vi "Calibration GUI.vi"(8 "error in (no error)":errorcluster, 9 "Skip Ref Mic":bool=TRUE, 10 "DB File":path, 11 "File":T3) -> (0 "error out":errorcluster)   [LabVIEW 2018]
uses:
  Types/EnumCalibration.ctl
  Microfontest/Peiker_Stepped Sweep Settings.ctl
  <vilib>/addons/_NISVFA/_Shared subVIs/Controls/svc_DSA Channel Settings.ctl
  <vilib>/addons/_NISVFA/_Shared subVIs/Controls/svc_Channel Info.ctl
  <vilib>/addons/_NISVFA/_Shared subVIs/Controls/svc_Engineering Units Text Ring.ctl
  <vilib>/addons/_NISVFA/_Shared subVIs/Controls/svc_Weighting Filter Text Ring.ctl
  <vilib>/Utility/file.llb/Read Delimited Spreadsheet (DBL).vi
  <vilib>/Utility/file.llb/Write Delimited Spreadsheet (DBL).vi
panel:
  in  "Error":string
  out "Model":bool
  in  "Terminate":bool
  in  "IAI Cal":bool
  in  "IAI Ret":bool
  in  "Cal Mic CH":bool
  out "Enum":T1
  in  "Ref mic value":dbl=4.2
  out "FrequencyList Level":T2(graph)
  out "Fundamental-Response":T4(graph)
  out "calibrated sensor sensitivity [mV/Pa]":dbl=nan format="%.2g"
  out "Reference Mic Power Spectrum":cluster{"x0":dbl, "dx":dbl, "magnitude":dbl[]}(graph)
  in  "Calibration Setting":T5={"Calibration Value (db SPL)"=94.0, "Calibration Frequency (Hz)"=1000.0}
  in  "Start":bool
  in  "Cancel Button":bool
  # "Calibration"
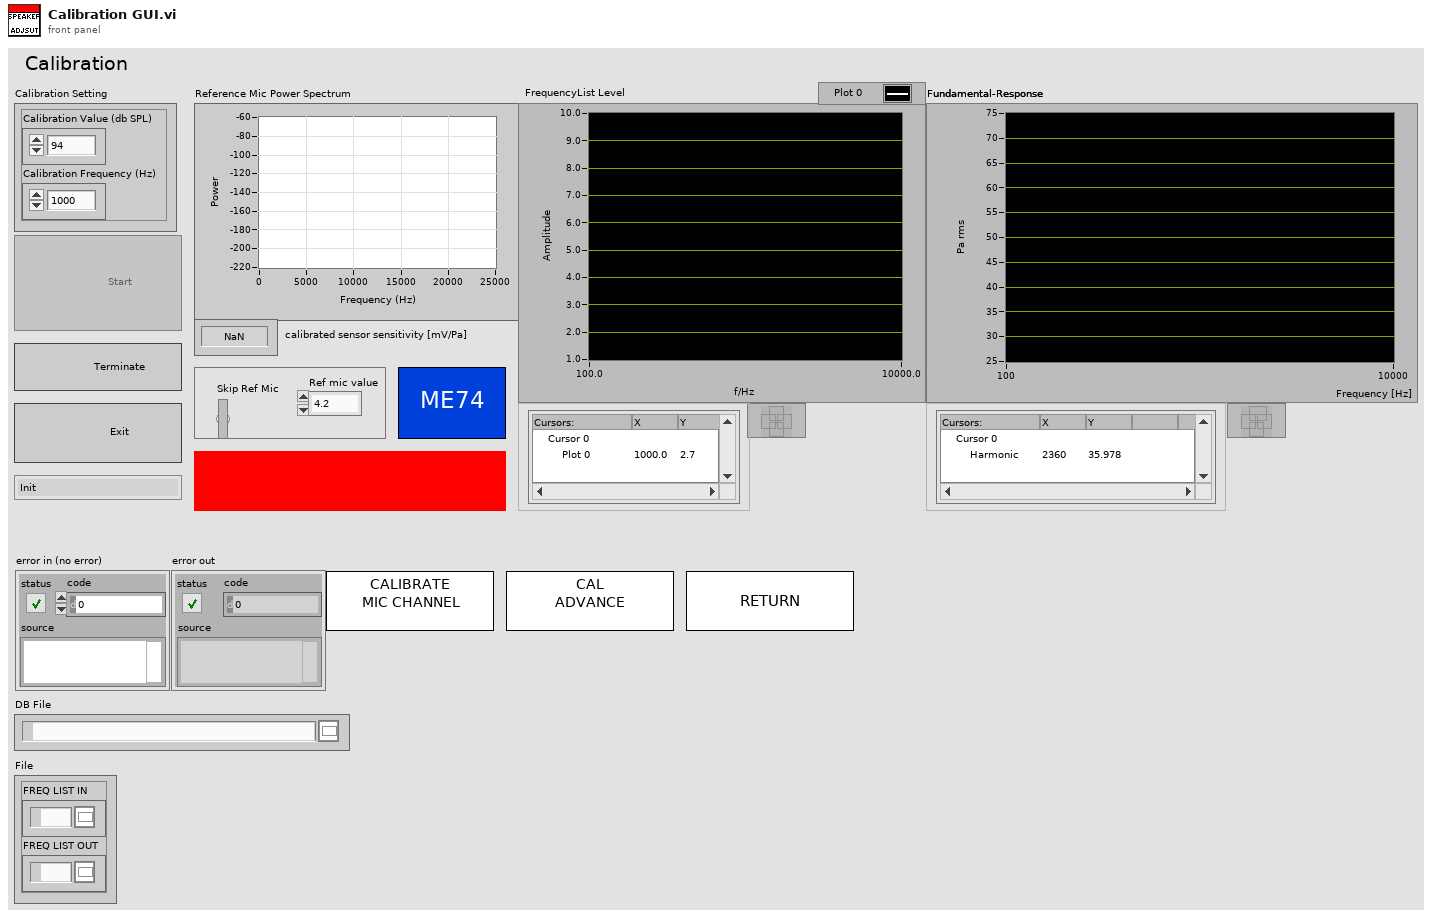
[diagram p1: front panel]
types:
  T1 = typedef "EnumCalibration.ctl" = enum16{"Init", "Idle", "IAI Return", "IAI Advance", "Read Reference Mic", "Adjust Speaker", "Save Adjustment Level", "Read Frequency", "Quit"}
  T2 = cluster{"frequency [Hz]":dbl, "amplitude [V]":dbl}[]
  T3 = cluster{"FREQ LIST IN":path, "FREQ LIST OUT":path}
  T4 = cluster{"frequency [Hz]":dbl[], "amplitude":dbl[]}
  T5 = cluster{"Calibration Value (db SPL)":dbl, "Calibration Frequency (Hz)":dbl}
  T6 = cluster{"SollPegel[dBSPL]":i32, "maxDeviationRef[dB]":dbl, "maxDeviation[dB]":dbl, "maxRuns":i32, "RefFrequency[Hz]":i32, "Wait[ms]":i32}
  T7 = typedef "Peiker_Stepped Sweep Settings.ctl" = cluster{"Input Settings":cluster{"IEPE min time to settle [s]":dbl, "Responce Channel Settings":cluster{"DSA response channel settings":T8, "response channel info":T9, "AI response settings":cluster{"response channel":tag, "max value [V]":dbl, "min value [V]":dbl, "terminal configuration":i32}}, "Stimulus Channel Settings":cluster{"AI stimulus settings":cluster{"stimulus channel":tag, "max value [V]":dbl, "min value [V]":dbl, "terminal configuration":i32}, "DSA stimulus channel settings":T8, "stimulus channel info":T9}}, "Output Settings":cluster{"AO source settings":cluster{"excitation channel":tag, "max value [V]":dbl, "min value [V]":dbl, "terminal configuration":i32}}}
  T8 = typedef "svc_DSA Channel Settings.ctl" = cluster{"coupling":i32, "enable IEPE excitation":bool, "IEPE current [mA]":dbl}
  T9 = typedef "svc_Channel Info.ctl" = cluster{"sensor sensitivity":dbl, "engineering units":T10, "dB reference":dbl, "custom label":string, "weighting filter":T11, "pregain":dbl}
  T10 = typedef "svc_Engineering Units Text Ring.ctl" = u16
  T11 = typedef "svc_Weighting Filter Text Ring.ctl" = u16
  T12 = cluster{"settle time [s]":dbl, "settle cycles":i32}
  T13 = enum8{"Enabled", "Disabled", "Disabled and Grayed Out"}
  T14 = enum16{"Left Button", "Center Button", "Right Button", "Window Close"}
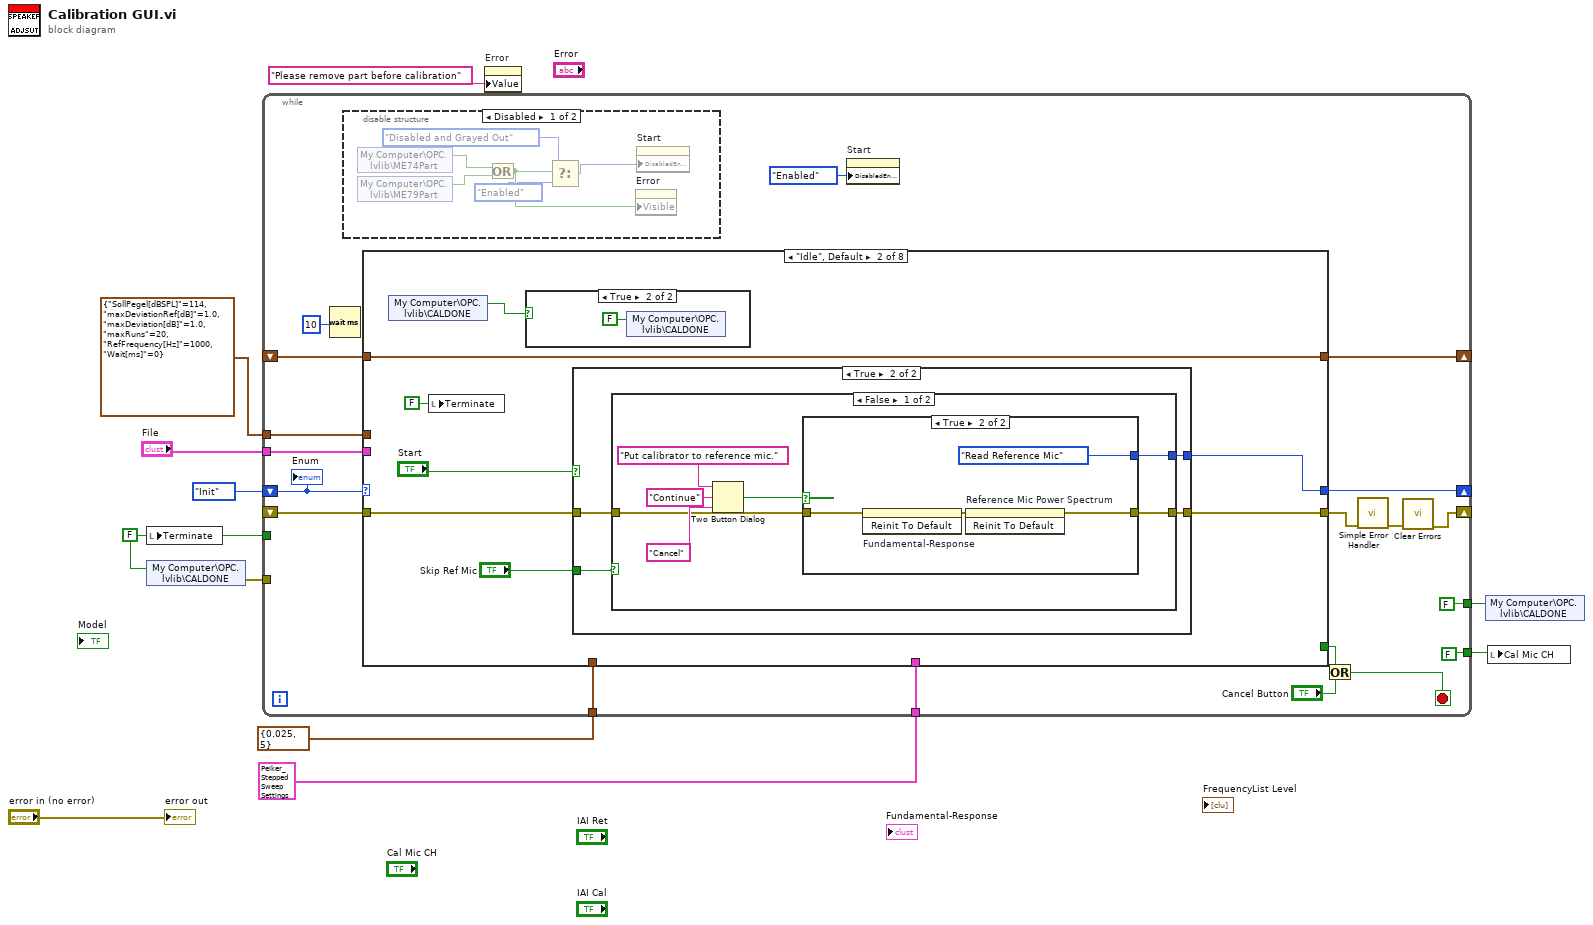
[diagram p0: block diagram]
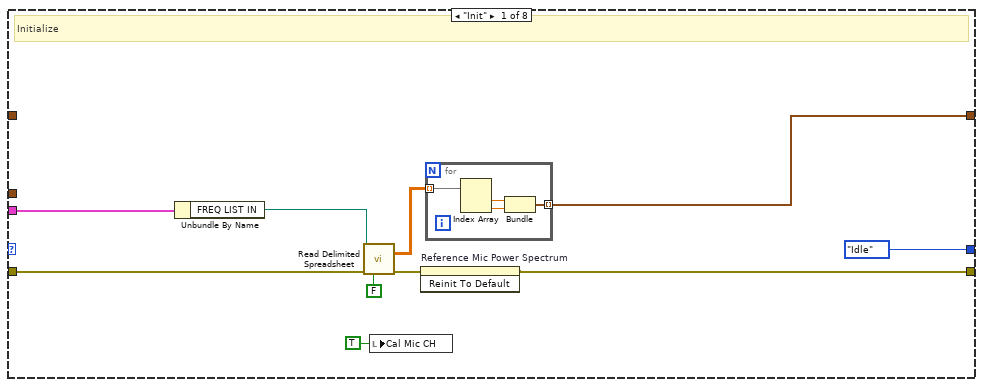
[diagram p3: hidden frame]
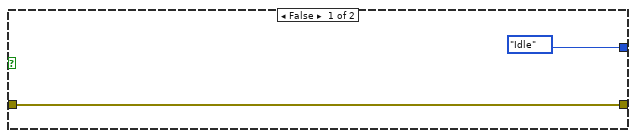
[diagram p5: hidden frame]
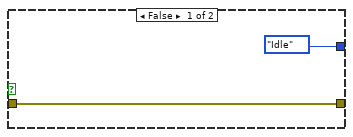
[diagram p6: hidden frame]
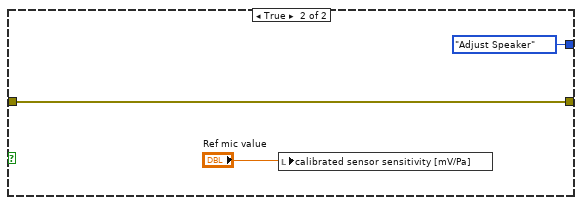
[diagram p7: hidden frame]
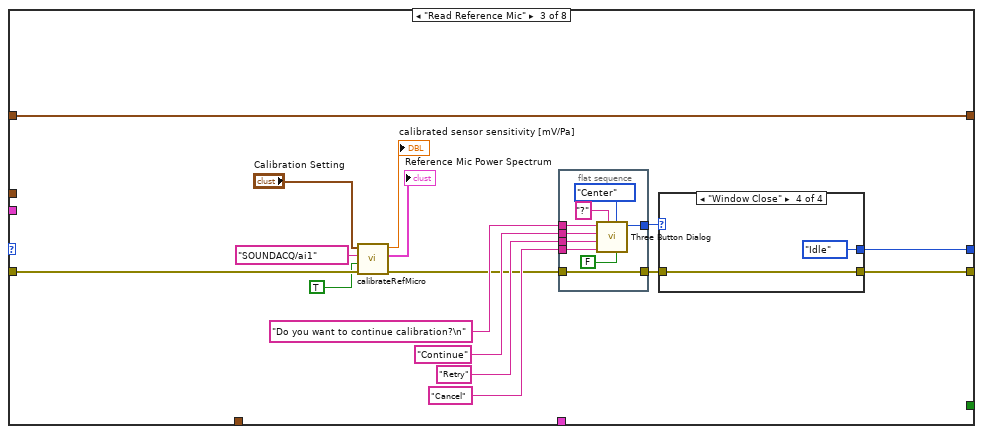
[diagram p8: hidden frame]
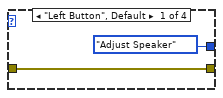
[diagram p9: hidden frame]
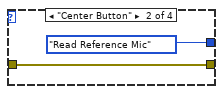
[diagram p10: hidden frame]
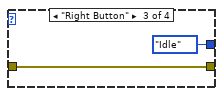
[diagram p11: hidden frame]
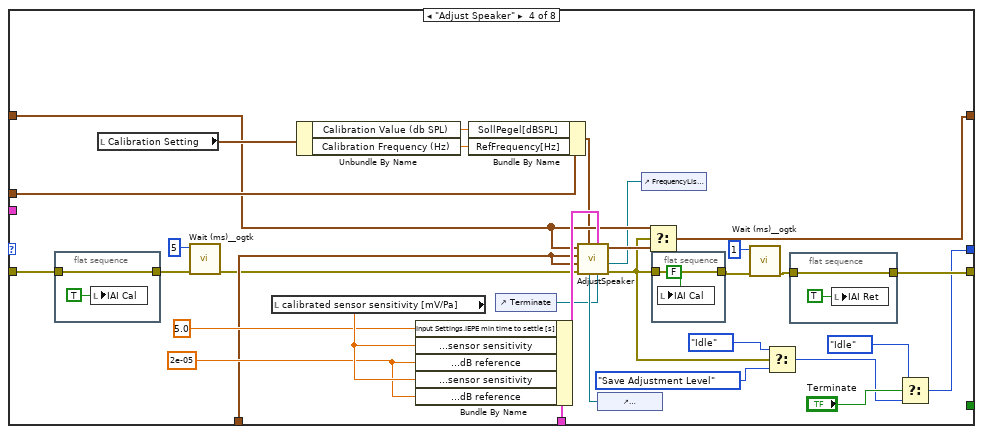
[diagram p12: hidden frame]
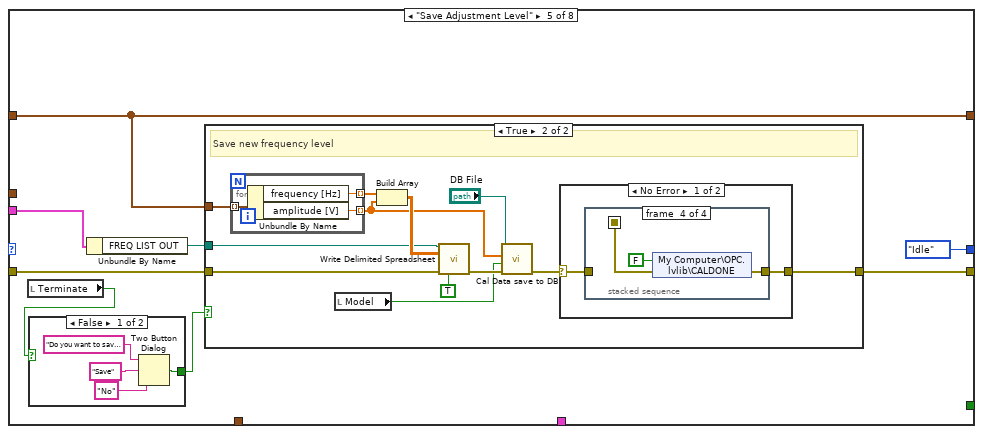
[diagram p13: hidden frame]
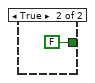
[diagram p14: hidden frame]
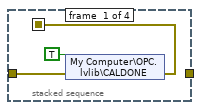
[diagram p16: hidden frame]
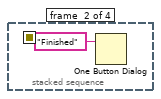
[diagram p17: hidden frame]
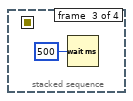
[diagram p18: hidden frame]
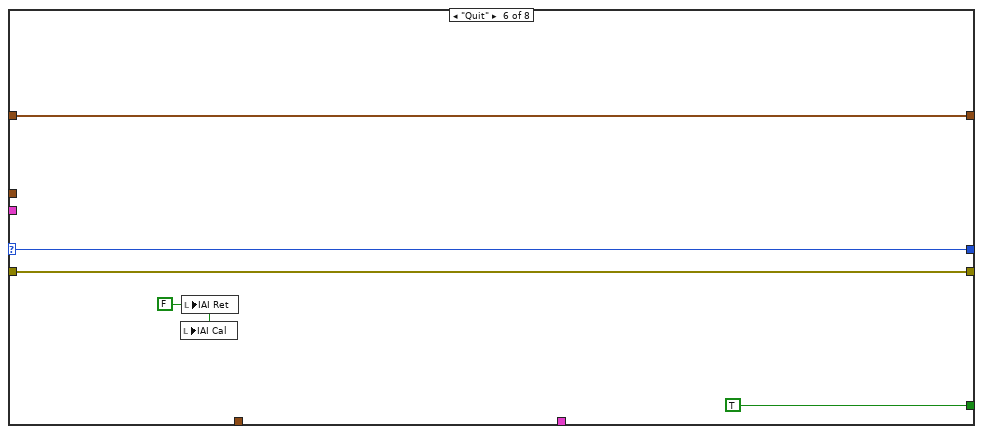
[diagram p20: hidden frame]
diagram:
  w3 = FALSE ("Terminate")
  n1 = local write "Terminate"(w3) -> ()
  n2 = shared-variable "My Computer\\OPC.lvlib\\CALDONE"(w3) -> (error out=w2:errorcluster)  [unwired: 1 in]
  n3 = while {
    shift-right: [w28] -> _
    shift-left: EnumCalibration."Init" -> [w30]
    shift-right: [w20] -> _
    shift-left: _ -> [w24]
    shift-right: [w23] -> _
    shift-left: _ -> [w19]
    tunnel: T12 {"settle time [s]"=0.025, "settle cycles"=5} ("settling time") -> [w18]
    tunnel: T6 {"SollPegel[dBSPL]"=114, "maxDeviationRef[dB]"=1.0, "maxDeviation[dB]"=1.0, "maxRuns"=20, "RefFrequency[Hz]"=1000, "Wait[ms]"=0} ("CalSettings") -> [w17]
    tunnel: T7 {"Input Settings"={"IEPE min time to settle [s]"=0.0, "Responce Channel Settings"={"DSA response channel settings"={"coupling"=10045, "enable IEPE excitation"=TRUE, "IEPE current [mA]"=4.0}, "response channel info"={"sensor sensitivity"=200.0, "engineering units"=2, "dB reference"=2e-05, "custom label"="EU", "weighting filter"=0, "pregain"=0.0}, "AI response settings"={"response channel"="SOUNDACQ/ai1", "max value [V]"=10.0, "min value [V]"=-10.0, "terminal configuration"=-1}}, "Stimulus Channel Settings"={"AI stimulus settings"={"stimulus channel"="SOUNDACQ/ai0", "max value [V]"=10.0, "min value [V]"=-10.0, "terminal configuration"=-1}, "DSA stimulus channel settings"={"coupling"=10045, "enable IEPE excitation"=FALSE, "IEPE current [mA]"=4.0}, "stimulus channel info"={"sensor sensitivity"=11.4, "engineering units"=2, "dB reference"=2e-05, "custom label"="EU", "weighting filter"=0, "pregain"=0.0}}}, "Output Settings"={"AO source settings"={"excitation channel"="SOUNDACQ/ao0", "max value [V]"=10.0, "min value [V]"=-10.0, "terminal configuration"=-1}}} ("Peiker_Stepped Sweep Settings") -> [w16]
    tunnel: "File" -> [w15]
    tunnel: [FALSE ("Cal Mic CH")] -> w5
    tunnel: w3 -> [_]
    tunnel: [FALSE ("CALDONE")] -> w4
    tunnel: w2 -> [_]
    stop <- w25 stop-if-true
    n4 = Wait (ms)(milliseconds to wait=u32 10) -> ()  [unwired: 1 out]
    n5 = disable-structure shown="Disabled" {
      frame Disabled {
        n6 = shared-variable "My Computer\\OPC.lvlib\\ME74Part"() -> (w36:bool)  [unwired: 1 in, 1 out]
        n7 = shared-variable "My Computer\\OPC.lvlib\\ME79Part"() -> (w35:bool)  [unwired: 1 in, 1 out]
        n8 = Or(x=w36, y=w35) -> (x .or. y?=w34:bool)
        n9 = Select(t=T13."Disabled and Grayed Out" ("Disabled"), s=w34, f=T13."Enabled" ("Disabled")) -> (s? t:f=w31:T13)
        n10 = property on="Error" class="Str"("Visible"=w34) -> ()  [unwired: 2 in, 2 out]
        n11 = property on="Start" class="Bool"("DisabledEnum"=w31) -> ()  [unwired: 2 in, 2 out]
      }
      frame Enabled {
      }
    }
    n12 = case shown="\"Idle\", Default" w30 {
      selector: w30 -> [_ _ _ _ _ w194 _ _]
      tunnel: [EnumCalibration."Idle" w54 w91 w115 EnumCalibration."Idle" w194 EnumCalibration."Init" EnumCalibration."Init"] -> w28
      tunnel: [_ _ _ _ _ TRUE _ _] -> w27
      tunnel: [w40 w55 w82 w120 w154 w195 w200 w203] -> w22
      tunnel: w24 -> [w43 w56 w97 w128 w160 w195 w200 w203]
      tunnel: [w42 w58 w96 w135 w159 w196 w198 w201] -> w23
      tunnel: w19 -> [_ w58 w96 w137 w159 w196 w198 w201]
      tunnel: w18 -> [_ _ _ w131 _ _ _ _]
      tunnel: w17 -> [_ _ _ w145 _ _ _ _]
      tunnel: w16 -> [_ _ _ w143 _ _ _ _]
      tunnel: w15 -> [w39 _ _ _ w158 _ _ _]
      frame "Init" {
        # "Initialize"
        n13 = Unbundle By Name(w39) -> ("FREQ LIST IN"=w38:path)
        n14 = call-poly <vilib>:"Read Delimited Spreadsheet.vi"("file path (dialog if empty)"=w38, "error in (no error)"=w43, "transpose? (F)"=FALSE) -> ("all rows"=w44:dbl[][], "error out"=w41:errorcluster)  [unwired: 7 in, 4 out]
        n15 = local write "Cal Mic CH"(TRUE ("Cal Mic CH")) -> ()
        n16 = invoke on="Reference Mic Power Spectrum" class="WFGraph (strict)" method="Reinit To Default"(error in=w41) -> (error out=w40:errorcluster)  [unwired: 2 in, 2 out]
        n17 = for {
          tunnel: w44 -> [w50] mode=indexing
          tunnel: [w47] -> w42 mode=indexing
          n18 = Index Array(array=w50) -> (element #1=w49:dbl, element #2=w48:dbl)  [unwired: 2 in]
          n19 = Bundle("Numeric"=w49, "Numeric"=w48) -> (w47:cluster{"Numeric":dbl, "Numeric":dbl})  [unwired: 1 in]
        }
      }
      frame "Idle", Default {
        n20 = shared-variable "My Computer\\OPC.lvlib\\CALDONE"() -> (w51:bool)  [unwired: 1 in, 1 out]
        n21 = local write "Terminate"(FALSE ("Terminate")) -> ()
        n22 = case shown="True" w51 {
          frame False {
          }
          frame True {
            n23 = shared-variable "My Computer\\OPC.lvlib\\CALDONE"(FALSE ("CALDONE")) -> ()  [unwired: 1 in, 1 out]
          }
        }
        n24 = case shown="True" "Start" {
          tunnel: w56 -> [w61 w63]
          tunnel: [w61 w65] -> w55
          tunnel: [EnumCalibration."Idle" w64] -> w54
          tunnel: "Skip Ref Mic" -> [_ w62]
          frame False {
          }
          frame True {
            n25 = case shown="False" w62 {
              tunnel: [w72 w80] -> w65
              tunnel: [w67 EnumCalibration."Adjust Speaker"] -> w64
              tunnel: w63 -> [w66 w80]
              frame False {
                n26 = Two Button Dialog(message="Put calibrator to reference mic.", 1:"Cancel", 2:"Continue" ("T button name (\"OK\")")) -> (T button?=w68:bool)
                n27 = case shown="True" w68 {
                  tunnel: [w73 w77] -> w72
                  tunnel: [EnumCalibration."Idle" EnumCalibration."Read Reference Mic"] -> w67
                  tunnel: w66 -> [w73 w75]
                  frame False {
                  }
                  frame True {
                    n28 = invoke on="Fundamental-Response" class="XYGraph (strict)" method="Reinit To Default"(error in=w75) -> (error out=w78:errorcluster)  [unwired: 2 in, 2 out]
                    n29 = invoke on="Reference Mic Power Spectrum" class="WFGraph (strict)" method="Reinit To Default"(error in=w78) -> (error out=w77:errorcluster)  [unwired: 2 in, 2 out]
                  }
                }
              }
              frame True {
                n30 = local write "calibrated sensor sensitivity [mV/Pa]"("Ref mic value") -> ()
              }
            }
          }
        }
      }
      frame "Read Reference Mic" {
        n31 = call "calibrateRefMicro.vi"("error in (no error)"=w97, "enable IEPE excitation (F)"=TRUE, "DAQmx physical channel"=tag "SOUNDACQ/ai1", "calibration settings"="Calibration Setting") -> ("error out"=w85:errorcluster, "power spectrum"=→"Reference Mic Power Spectrum":cluster{"x0":dbl, "dx":dbl, "magnitude":dbl[]}, "calibrated sensor sensitivity [mV/Pa]"=→"calibrated sensor sensitivity [mV/Pa]":dbl)  [unwired: 5 in]
        n32 = flat-sequence {
          tunnel: w85 -> [w107]
          tunnel: "Do you want to continue calibration?\n" -> [w114]
          tunnel: "Continue" ("Left Button Text (\"Yes\")") -> [w113]
          tunnel: "Retry" ("Left Button Text (\"Yes\")") -> [w112]
          tunnel: "Cancel" ("Left Button Text (\"Yes\")") -> [w111]
          tunnel: [w107] -> w83
          tunnel: [w106] -> w84
          frame #0 {
            n33 = call <vilib>:"Three Button Dialog.vi"("Allow user to close window? (TRUE)"=FALSE, "Justify Message (Left)"=enum16{"Left", "Center", "Right"}."Center", "Window Title (\"\")"="?", "Right Button Text (\"Cancel\")"=w111, "Center Button Text (\"No\")"=w112, "Left Button Text (\"Yes\")"=w113, "message"=w114) -> ("Which Button?"=w106:T14)  [unwired: 4 in]
          }
        }
        n34 = case shown="\"Window Close\"" w84 {
          tunnel: [EnumCalibration."Adjust Speaker" EnumCalibration."Read Reference Mic" EnumCalibration."Idle" EnumCalibration."Idle"] -> w91
          tunnel: w83 -> [w98 w100 w102 w105]
          tunnel: [w98 w100 w102 w105] -> w82
          frame "Left Button", Default {
          }
          frame "Center Button" {
          }
          frame "Right Button" {
          }
          frame "Window Close" {
          }
        }
      }
      frame "Adjust Speaker" {
        w141 = 2e-05 ("Input Settings.Responce Channel Settings.response channel info.dB reference")
        n35 = flat-sequence {
          tunnel: w128 -> [w151]
          tunnel: [w151] -> w127
          frame #0 {
            n36 = local write "IAI Cal"(TRUE ("IAI Cal")) -> ()
          }
        }
        n37 = local read "Calibration Setting"() -> (w146:T5)
        n38 = call <userlib>:"Wait (ms)__ogtk.vi"("error in (no error)"=w127, "milliseconds to wait"=u32 5) -> ("error out"=w125:errorcluster)  [unwired: 8 in, 1 out]
        n39 = local read "calibrated sensor sensitivity [mV/Pa]"() -> (w142:dbl)
        n40 = Unbundle By Name(w146) -> ("Calibration Value (db SPL)"=w144:dbl, "Calibration Frequency (Hz)"=w134:dbl)
        n41 = Bundle By Name(cluster=w143, "Input Settings.IEPE min time to settle [s]"=5.0, "Input Settings.Responce Channel Settings.response channel info.sensor sensitivity"=w142, "Input Settings.Responce Channel Settings.response channel info.dB reference"=w141, "Input Settings.Stimulus Channel Settings.stimulus channel info.sensor sensitivity"=w142, "Input Settings.Stimulus Channel Settings.stimulus channel info.dB reference"=w141) -> (w140:T7)
        n42 = Bundle By Name(cluster=w145, "SollPegel[dBSPL]"=w144, "RefFrequency[Hz]"=w134) -> (w129:T6)
        n43 = control-ref of="Terminate"() -> (w119:refnum<vi>)
        n44 = control-ref of="Fundamental-Response"() -> (w138:refnum<vi>)
        n45 = control-ref of="FrequencyList Level"() -> (w130:refnum<vi>)
        n46 = call "AdjustSpeaker.vi"("Input Signal"=w130, "Terminate"=w119, "Peiker_Stepped Sweep Settings"=w140, "Fundamental Amplitude 2"=w138, "CalSettings"=w129, "error in"=w125, "integration time"=w131, "settling time"=w131, "Frequency List"=w137) -> ("error out"=w124:errorcluster, "correctedFreqList"=w136:T2)  [unwired: 1 out]
        n47 = Select(t=w137, s=w124, f=w136) -> (s? t:f=w135:T2)
        n48 = flat-sequence {
          tunnel: w124 -> [w149]
          tunnel: [w149] -> w122
          frame #0 {
            n49 = local write "IAI Cal"(FALSE ("IAI Cal")) -> ()
          }
        }
        n50 = call <userlib>:"Wait (ms)__ogtk.vi"("error in (no error)"=w122, "milliseconds to wait"=u32 1) -> ("error out"=w121:errorcluster)  [unwired: 8 in, 1 out]
        n51 = Select(t=EnumCalibration."Idle", s=w124, f=EnumCalibration."Save Adjustment Level") -> (s? t:f=w117:T1)
        n52 = flat-sequence {
          tunnel: w121 -> [w148]
          tunnel: [w148] -> w120
          frame #0 {
            n53 = local write "IAI Ret"(TRUE ("IAI Ret")) -> ()
          }
        }
        n54 = Select(t=EnumCalibration."Idle", s="Terminate", f=w117) -> (s? t:f=w115:T1)
      }
      frame "Save Adjustment Level" {
        n55 = local read "Terminate"() -> (w153:bool)
        n56 = case shown="False" w153 {
          tunnel: [w161 FALSE ("T button?")] -> w155
          frame False {
            n57 = Two Button Dialog(message="Do you want to save new frequency level?", 1:"No" ("F button name (\"Cancel\")"), 2:"Save" ("T button name (\"OK\")")) -> (T button?=w161:bool)
          }
          frame True {
          }
        }
        n58 = Unbundle By Name(w158) -> ("FREQ LIST OUT"=w157:path)
        n59 = case shown="True" w155 {
          tunnel: w160 -> [w166 w175]
          tunnel: w159 -> [_ w174]
          tunnel: [w166 w167] -> w154
          tunnel: w157 -> [_ w173]
          frame False {
          }
          frame True {
            # "Save new frequency level"
            n60 = for {
              tunnel: w174 -> [w192] mode=indexing
              tunnel: [w191] -> w177 mode=indexing
              tunnel: [w190] -> w170 mode=indexing
              n61 = Unbundle By Name(w192) -> ("frequency [Hz]"=w191:dbl, "amplitude [V]"=w190:dbl)
            }
            n62 = local read "Model"() -> (w169:bool)
            n63 = Build Array(w177, w170) -> (w178:dbl[][])
            n64 = call-poly <vilib>:"Write Delimited Spreadsheet.vi"("file path (dialog if empty)"=w173, "2D data"=w178, "error in (no error)"=w175, "transpose? (no:F)"=TRUE) -> ("error out"=w172:errorcluster)  [unwired: 10 in, 1 out]
            n65 = call "Cal Data save to DB.vi"("Error In"=w172, "Model (F-ME74)"=w169, "Adjusted Amplitude"=w170, "DB File"="DB File") -> ("Error Out"=w168:errorcluster)  [unwired: 7 in]
            n66 = case shown="No Error" w168 {
              selector: w168 -> [w180 w189]
              tunnel: [w179 w189] -> w167
              frame No Error {
                n67 = stacked-sequence {
                  seq-local: [w181 _ _ _] -> [_ _ _ w187]
                  tunnel: w180 -> [w183 _ _ _]
                  tunnel: [_ _ _ w186] -> w179
                  frame #0 {
                    n68 = shared-variable "My Computer\\OPC.lvlib\\CALDONE"(TRUE ("CALDONE"), error in=w183) -> (error out=w181:errorcluster)
                  }
                  frame #1 {
                    n69 = One Button Dialog(message="Finished") -> ()  [unwired: 1 in, 1 out]
                  }
                  frame #2 {
                    n70 = Wait (ms)(milliseconds to wait=u32 500) -> ()  [unwired: 1 out]
                  }
                  frame #3 {
                    n71 = shared-variable "My Computer\\OPC.lvlib\\CALDONE"(FALSE ("CALDONE"), error in=w187) -> (error out=w186:errorcluster)
                  }
                }
              }
              frame Error {
              }
            }
          }
        }
      }
      frame "Quit" {
        w193 = FALSE ("IAI Ret")
        n72 = local write "IAI Cal"(w193) -> ()
        n73 = local write "IAI Ret"(w193) -> ()
      }
      frame "IAI Return" {
      }
      frame "IAI Advance" {
      }
    }
    n74 = property on="Start" class="Bool"("DisabledEnum"=T13."Enabled" ("Disabled")) -> ()  [unwired: 2 in, 2 out]
    n75 = Or(x=w27, y="Cancel Button") -> (x .or. y?=w25:bool)
    n76 = call <vilib>:"Simple Error Handler.vi"("error in (no error)"=w22) -> ("error out"=w21:errorcluster)  [unwired: 4 in, 4 out]
    n77 = call <vilib>:"Clear Errors.vi"("error in (no error)"=w21) -> ("error out"=w20:errorcluster)  [unwired: 5 in, 1 out]
    "Enum" <- w30
  }
  n78 = property on="Error" class="Str"("Value"="Please remove part before calibration" ("Error")) -> ()  [unwired: 2 in, 2 out]
  n79 = shared-variable "My Computer\\OPC.lvlib\\CALDONE"(w4) -> ()  [unwired: 1 in, 1 out]
  n80 = local write "Cal Mic CH"(w5) -> ()
  "error out" <- "error in (no error)"
